vi "Init Node.vi"(7 "Launch Events":bool, 8 "error in (no error)":errorcluster, 11 "Volatus Core in":refnum<class "Volatus Core.lvclass">) -> (0 "error out":errorcluster, 3 "Volatus Core out":refnum<class "Volatus Core.lvclass">)   [LabVIEW 2020, in "Volatus.lvlib" / "Volatus Core.lvclass"]
uses:
  Volatus Core.lvclass
  C:/dev/lv20CE/relink/lv-volatus/Volatus/Module/Module.lvclass
  Module/Module.lvclass/Module.ctl
  Volatus Core.lvclass/Volatus Core.ctl
  MessageQ/MessageQ.lvclass/MessageQ.ctl
  MessageQ/Send.vi
  Module/Module.lvclass
  VolatusAPI/VolatusAPI.lvclass
  C:/dev/lv20CE/relink/lv-volatus/Volatus/Volatus Core/Volatus Core.lvclass
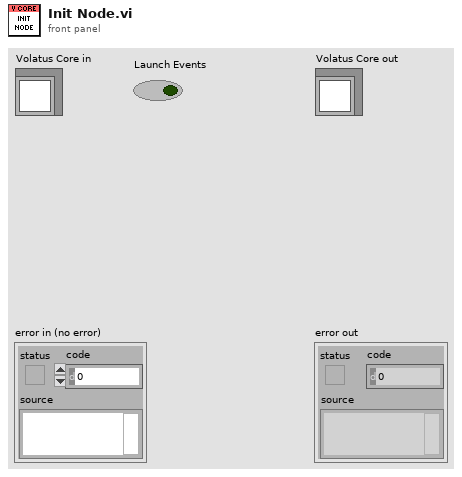
[diagram p1: front panel]
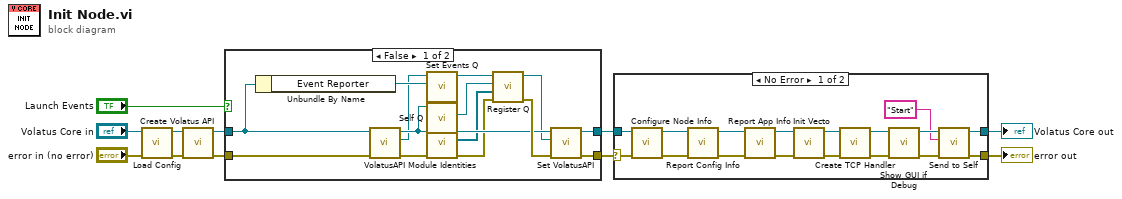
[diagram p0: block diagram]
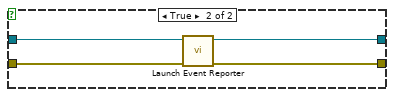
[diagram p2: hidden frame]
diagram:
  n1 = call "Load Config.vi"("error in (no error)"="error in (no error)", "Volatus Core in"="Volatus Core in") -> ("error out"=w11:errorcluster, "Volatus Core out"=w10:refnum<class "Volatus Core.lvclass">)  [unwired: 8 in]
  n2 = call "Create Volatus API.vi"("error in (no error)"=w11, "Volatus Core in"=w10) -> ("error out"=w5:errorcluster, "Volatus Core out"=w4:refnum<class "Volatus Core.lvclass">)  [unwired: 8 in]
  n3 = case shown="False" "Launch Events" {
    tunnel: w5 -> [w12 w28]
    tunnel: w4 -> [w13 w26]
    tunnel: [w24 w27] -> w1
    tunnel: [w14 w25] -> w2
    frame False {
      n4 = Unbundle By Name(w13) -> ("Event Reporter"=w23:refnum<class "MessageQ.lvclass">)
      n5 = call "VolatusAPI.vi"("Module in"=w13) -> ("VolatusAPI"=w15:refnum<class "VolatusAPI.lvclass">, "Module out"=w18:refnum<class "Volatus Core.lvclass">)  [unwired: 9 in]
      n6 = call "Set Events Q.vi"("Events Q"=w23, "VolatusAPI in"=w15) -> ("VolatusAPI out"=w16:refnum<class "VolatusAPI.lvclass">)  [unwired: 9 in]
      n7 = call "Self Q.vi"("Module in"=w18) -> ("Self Q"=w19:refnum<class "MessageQ.lvclass">)  [unwired: 9 in, 1 out]
      n8 = call-dynamic "Module Identities.vi"("error in (no error)"=w12, "Volatus Core in"=w18) -> ("error out"=w20:errorcluster, "Identities"=w17:refnum<class "Identity.lvclass">[], "Volatus Core out"=w22:refnum<class "Volatus Core.lvclass">)  [unwired: 7 in]
      n9 = call "Register Q.vi"("error in (no error)"=w20, "Identities"=w17, "MessageQ"=w19, "VolatusAPI in"=w16) -> ("error out"=w24:errorcluster, "VolatusAPI out"=w21:refnum<class "VolatusAPI.lvclass">)  [unwired: 5 in, 1 out]
      n10 = call "Set VolatusAPI.vi"("VolatusAPI"=w21, "Module in"=w22) -> ("Module out"=w14:refnum<class "Volatus Core.lvclass">)  [unwired: 9 in]
    }
    frame True {
      n11 = call "Launch Event Reporter.vi"("error in (no error)"=w28, "Volatus Core in"=w26) -> ("error out"=w27:errorcluster, "Volatus Core out"=w25:refnum<class "Volatus Core.lvclass">)  [unwired: 8 in]
    }
  }
  n12 = case shown="No Error" w1 {
    selector: w1 -> [w45 w46]
    tunnel: w2 -> [w32 w47]
    tunnel: [w38 w47] -> w7
    tunnel: [w40 w46] -> w6
    frame No Error {
      n13 = call "Configure Node Info.vi"("error in (no error)"=w45, "Volatus Core in"=w32) -> ("error out"=w33:errorcluster, "Volatus Core out"=w30:refnum<class "Volatus Core.lvclass">)  [unwired: 8 in]
      n14 = call "Report Config Info.vi"("error in (no error)"=w33, "Volatus Core in"=w30) -> ("error out"=w31:errorcluster, "Volatus Core out"=w29:refnum<class "Volatus Core.lvclass">)  [unwired: 8 in]
      n15 = call "Report App Info.vi"("error in (no error)"=w31, "Volatus Core in"=w29) -> ("error out"=w44:errorcluster, "Volatus Core out"=w41:refnum<class "Volatus Core.lvclass">)  [unwired: 8 in]
      n16 = call "Init Vecto.vi"("error in (no error)"=w44, "Volatus Core in"=w41) -> ("error out"=w42:errorcluster, "Volatus Core out"=w35:refnum<class "Volatus Core.lvclass">)  [unwired: 8 in]
      n17 = call "Create TCP Handler.vi"("error in (no error)"=w42, "Volatus Core in"=w35) -> ("error out"=w36:errorcluster, "Volatus Core out"=w34:refnum<class "Volatus Core.lvclass">)  [unwired: 8 in]
      n18 = call "Show GUI if Debug.vi"("error in (no error)"=w36, "Module in"=w34) -> ("error out"=w43:errorcluster, "Module out"=w39:refnum<class "Volatus Core.lvclass">)  [unwired: 8 in]
      n19 = call "Send to Self.vi"("error in (no error)"=w43, "Message ID"="Start", "Module in"=w39) -> ("error out"=w40:errorcluster, "Module out"=w38:refnum<class "Volatus Core.lvclass">)  [unwired: 7 in]
    }
    frame Error {
    }
  }
  "error out" <- w6
  "Volatus Core out" <- w7
